vi "Extract Element JSON.vi"(11 "Ctl Refnum in":refnum<vi>) -> (0 "JSON":string, 1 "Type":string, 2 "Is GUI Element":bool, 3 "Ctl Refnum":refnum<vi>)   [LabVIEW 2020, in "VolatusGUI.lvlib"]
uses:
  VolatusGUI.lvlib
  <vilib>/JDP Science/JSONtext/JSONtext.lvlib
  74616f74-1830-4ff5-a2b6-8e366ce61fd3.vi
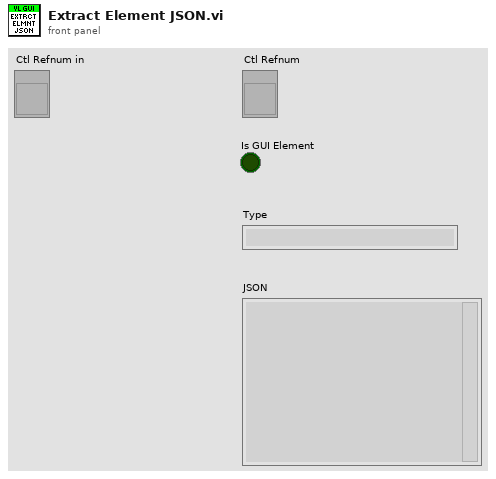
[diagram p1: front panel]
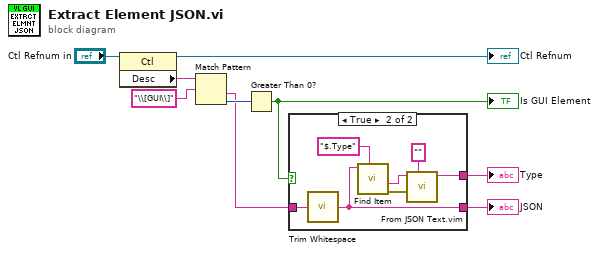
[diagram p0: block diagram]
diagram:
  n1 = property class="Ctl"(reference="Ctl Refnum in") -> (reference out=→"Ctl Refnum":refnum<vi>, "Desc"=w9:string)  [unwired: 1 in, 1 out]
  n2 = Match Pattern(string=w9, regular expression="\\[GUI\\]") -> (after substring=w3:string, offset past match=w7:i32)  [unwired: 1 in, 2 out]
  n3 = Greater Than 0?(x=w7) -> (x > 0?=w4:bool)
  "Is GUI Element" <- w4
  n4 = case shown="True" w4 {
    tunnel: w3 -> [_ w16]
    tunnel: [_ w11] -> w2
    tunnel: [_ w10] -> w1
    frame False {
    }
    frame True {
      n5 = call <vilib>:"Trim Whitespace.vi"("string"=w16) -> ("trimmed string"=w10:string)  [unwired: 1 in]
      n6 = call <vilib>:"Find Item.vi"("$Path or Item Name"="$.Type", "JSON"=w10) -> ("error out"=w14:errorcluster, "<JSON>"=w13:string)  [unwired: 6 in, 2 out]
      n7 = call "From JSON Text.vim"("Data Type and Default Value"="", "error in (no error)"=w14, "JSON"=w13) -> ("Data out"=w11:string)  [unwired: 7 in, 1 out]
    }
  }
  "Type" <- w2
  "JSON" <- w1
